vi "AddRequest.vi"(8 "error in (no error)":errorcluster, 10 "Request":string, 11 "Room Number":i32) -> (0 "error out":errorcluster, 2 "Response":string)   [LabVIEW 2015, in "RestApi.lvlib"]
uses:
  RestApi.lvlib
  TypeDef/PostRoomCommands.ctl
panel:
  out "JSON string":string
  # "{\"FlagsState\":\"{\\\"State\\\":[false,false,false,false],\\\"Color\\\":[0,1,2,3]}\"}"
  # "http://127.0.0.1:8001/WebService1/UpdateFlagState?Room={value}&FlagState={value}"
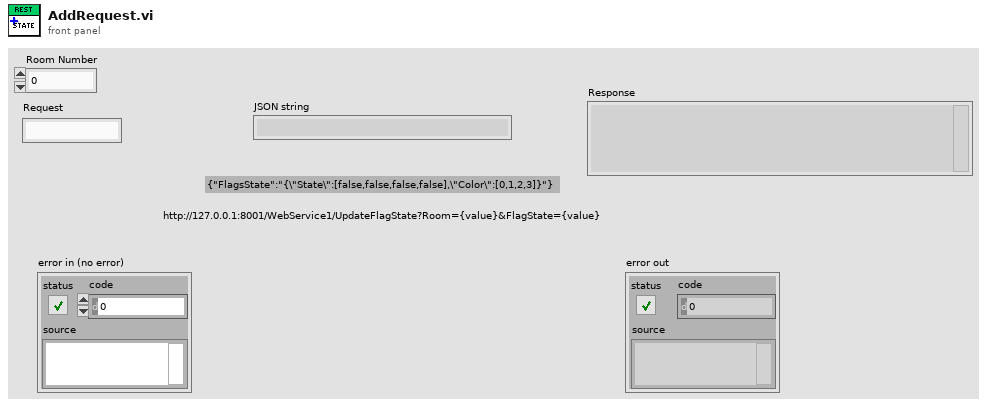
[diagram p1: front panel]
types:
  T1 = typedef "RestApi.lvlib/PostRoomCommands.ctl" = enum16{"WriteFlagState", "WriteFlagColor", "WriteBedVacant", "AddPersonnel", "RemovePersonnel", "AddRequest", "RemoveRequest", "WriteBeaconID", "WriteBedURL"}
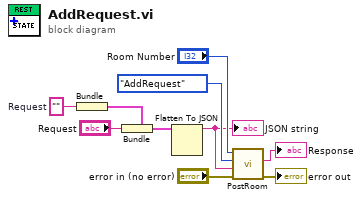
[diagram p0: block diagram]
diagram:
  w4 = ""  # Request
  n1 = Bundle("Request"=w4) -> (w3:cluster{"Request":string})  [unwired: 1 in]
  n2 = Bundle(cluster=w3, "Request"="Request") -> (w2:cluster{"Request":string})
  n3 = Flatten To JSON(anything=w2) -> (JSON string=w5:string)  [unwired: 2 in, 1 out]
  "JSON string" <- w5
  n4 = call "PostRoom.vi"("error in (no error)"="error in (no error)", "Data"=w5, "Enum"=PostRoomCommands."AddRequest", "Room Number"="Room Number") -> ("error out"=→"error out":errorcluster, "body"=→"Response":string)  [unwired: 6 in]
